vi "Generation Example.vi"() -> ()   [LabVIEW 2025, in "GettingStarted_Gen_148X_Host.lvlib"]
uses:
  GettingStarted_Gen_148X_Host.lvlib
  Common/Types/Serial Channel Configuration.ctl
  <instrlib>/FlexRIO/CSI-2/v2/FPGA/Types/Display Parameters.ctl
  <instrlib>/FlexRIO/CSI-2/v2/Common/Types/LLP Data Type.ctl
  Common/Types/RAW Interpretation for Display.ctl
  <vilib>/userDefined/Silver/nirio_resource_slv.ctl
  <instrlib>/FlexRIO/CSI-2/v2/FPGA/Types/Timestamp ID.ctl
  Common/Types/GPIO Filter.ctl
  Common/Types/Packet Table.ctl
  FPGA/Common/Types/SerDes Identifier.ctl
  <instrlib>/FlexRIO/CSI-2/v2/FPGA/Types/GPIO Bank.ctl
  Common/Types/GPIO Route Configuration.ctl
  Common/Types/GPIO Route Direction.ctl
  Common/Types/GPIO Route Line.ctl
  <vilib>/vision/Image Controls.llb/IMAQ Image.ctl
  <vilib>/Utility/miscctls.llb/LVRowAndColumnUnsignedTypeDef.ctl
  <instrlib>/FlexRIO/API/Host/v1/NI FlexRIO/API/Wait for PoC Safe to Disconnect Channels Array.vi
  <vilib>/FPGAPlugInAG/Dynamic/niLvFpga_Close_Dynamic.vi
  <vilib>/rvi/interface/nirviCloseFPGA/nirviCloseFPGA.xnode
  <instrlib>/FlexRIO/API/Host/v1/NI FlexRIO API v1.lvlib
  Common/GettingStarted_Common_148X_Host.lvlib
  <instrlib>/FlexRIO/CSI-2/v2/FPGA/NI CSI-2 API FPGA v2.lvlib
  FPGA/Common/GettingStarted_Common_148X_FPGA.lvlib
  <instrlib>/FlexRIO/CSI-2/v2/Common/NI CSI-2 API Common v2.lvlib
panel:
  out "Power Over Coax Source In Range":bool[](array[boolean])
  in  "Configuration":T1(tab)
  in  "Display Generated Images":bool=TRUE
  in  "RIO Device":T2="PXI1Slot5"
  in  "Bitfile Path":path=path "C:/dev/hardware-validation/src/labview/auto-vision/Automotive Vision/1487 HIHO GSE/FPGA Bitfiles/PXIe_1487_4_In_4_Out_Gen.lvbitx"
  in  "TDMS File Directory":path=path "C:/dev/hardware-validation/src/labview/auto-vision/Automotive Vision/1487 HIHO GSE/TDMS800x600raw8"
  in  "Log I2C to Disk":bool
  in  "Log GPIO to Disk":bool
  in  "Channel Configurations":T3[](array[typedef])=[{"Serial Channel"="SO1", "FPGA Display Parameters"={"virtual channel"=0.0, "payload data type"=enum."RAW 8", "frame skip count"=0, "line skip count"=0, "pixel skip count"=0.0}, "RAW Display Parameters"={"Interpretation"=enum."Bayer", "Bayer Parameters"={"Pattern"=3, "Algorithm"=0, "Red Gain"=1.0, "Green Gain"=1.0, "Blue Gain"=1.0}}}] {"RAW Display Parameters"."Bayer Parameters"."Blue Gain" min=0.0 max=3.99 step=0.1 format="%_4g"; "RAW Display Parameters"."Bayer Parameters"."Green Gain" min=0.0 max=3.99 step=0.1 format="%_4g"; "RAW Display Parameters"."Bayer Parameters"."Red Gain" min=0.0 max=3.99 step=0.1 format="%_4g"; "RAW Display Parameters"."Bayer Parameters"."Algorithm" items=["Bilinear", "VNG"]; "RAW Display Parameters"."Bayer Parameters"."Pattern" items=["GB", "GR", "BG", "RG"]}
  in  "Serializer (Output) Configuration Script":path=path "C:/dev/hardware-validation/src/labview/auto-vision/Automotive Vision/1487 HIHO GSE/scripts/Image RT Scripts/9295A_RAW8.cpp"
  in  "Packet Timing Error Threshold (s)":dbl=1e-06 format="%#_6p"
  in  "Start Trigger Delay (s)":dbl min=0.0
  out "Actual Serial Output Data Rate (bps)":dbl=-1.0 format="%#_6p"
  in  "Power Over Coax Sink":i32(ring) items=["None"=0, "Auxiliary"=2]
  in  "Reference Clock Frequency (Hz)":dbl=25000000.0 format="%#_6p"
  in  "Requested Serial Ouptut Data Rate (bps)":dbl=-1.0 format="%#_6p"
  in  "Serial Output Active Lane Count":i32(ring)=4 items=["1 Lane"=1, "2 Lanes"=2, "4 Lanes"=4]
  in  "Power Over Coax Source":i32(ring) items=["None", "Internal", "Auxiliary"]
  in  "Timestamp Filter":T7[](array[typedef])
  in  "Enable I2C TAP (All Channels)":bool=TRUE
  in  "GPIO Bank Output Enable":T8
  in  "GPIO Routes":T9[](array[typedef]) {"Serial Channel" max=3 step=1}
  in  "GPIO to Display":T12[](array[typedef])
  in  "GPIO Bank Select":T13
  in  "GPIO Bank Output":T8
  out "GPIO Bank Read":T8
  in  "Update GPIO Output":bool
  in  "Generated Serial Output Channel Data":T14(tab)
  out "Source Rate (fps)(1st Display)":dbl
  out "Update Rate (fps)(1st Display)":dbl
  in  "Serial Channel (1st Display)":fxp<+,3,3>
  out "1st channel display":T15(plugin-control)
  out "Source Rate (fps)(2nd Display)":dbl
  out "Update Rate (fps)(2nd Display)":dbl
  out "2nd channel display":T15(plugin-control)
  in  "Serial Channel (2nd Display)":fxp<+,3,3>
  out "I2C Timestamps":T16
  out "GPIO Timestamps Waveform":digitalwaveform[](graph)
  out "Error Parsing GPIO Timestamps":bool
  out "Generation State":T17(ring)
  out "Number of Generated Packets":u64[](array[numeric])
  out "Packet Timing Errors":bool[](array[boolean])
  out "Waiting for Serializer Setup":bool
  in  "Serializer Setup Complete":bool
  out "Generation Stopped":bool
  out "Power Over Coax Voltage (V)":dbl[](array[numeric]) format="%#.2pV"
  out "Power Over Coax Current (A)":dbl[](array[numeric]) format="%#.2pA"
  out "Power Over Coax Sink In Range":bool[](array[boolean])
  in  "Stop Generation":bool
  out "Error Out":errorcluster
  # "Overview: Configure a generation to replay CSI-2 data and timestamps from disk.\nInstructions: Visit https://ni.com/r/automotive-camera-module-ref for tutorials and reference material on using this example with the PXIe-148X."
  # "Configuration Settings"
  # "Data Output"
  # "Note: Applies to Tap Boards only with\nI2C -> Enable I2C TAP (All Channels) enabled"
  # "Resource Configuration"
  # "Output Configuration"
  # "Channel Configuration"
  # "Power Over Coax Configuration"
  # "Note: Applies to Tap Boards only with\nI2C -> Enable I2C TAP (All Channels) enabled"
  # "Clocking Configuration"
  # "CSI-2 Output Configuration"
  # "Use -1 to request the default data rate"
  # "I2C Timestamp Configuration"
  # "The timestamp filters listed correspond to the I2C traffic for a specific serial channel:\n\nUser24 = SO0\nUser25 = SO1\nUser26 = SO2\nUser27 = SO3\nUser28 = SO4\nUser29 = SO5\nUser30 = SO6\nUser31 = SO7"
  # "I2C TAP Configuration (4 In/4 Out Only)"
  # "GPIO Display Configuration"
  # "GPIO Bank Read / Write Configuration"
  # "GPIO Routing Configuration"
  # "NOTE: Image Display is currently only supported on Windows."
  # "NOTE: Image Display is currently only supported on Windows."
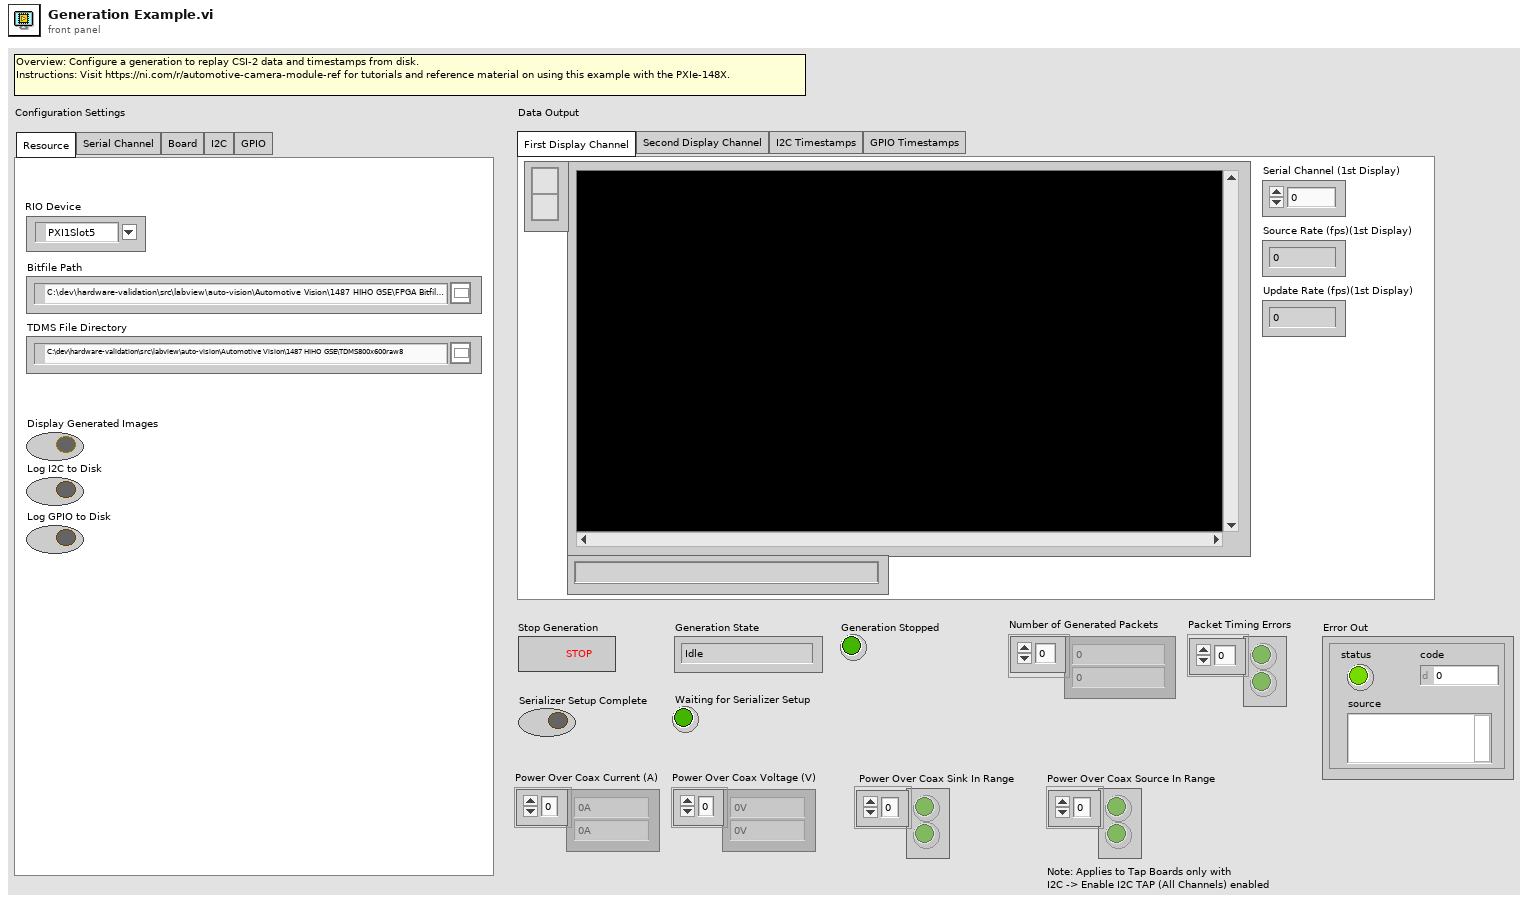
[diagram p1: front panel]
types:
  T1 = enum32{"Resource", "Serial Channel", "Board", "I2C", "GPIO"}
  T2 = typedef "nirio_resource_slv.ctl" = tag
  T3 = typedef "GettingStarted_Common_148X_Host.lvlib/Serial Channel Configuration.ctl" = cluster{"Serial Channel":string, "FPGA Display Parameters":T4, "RAW Display Parameters":cluster{"Interpretation":T6, "Bayer Parameters":cluster{"Pattern":i32, "Algorithm":i32, "Red Gain":dbl, "Green Gain":dbl, "Blue Gain":dbl}}}
  T4 = typedef "NI CSI-2 API FPGA v2.lvlib/Display Parameters.ctl" = cluster{"virtual channel":fxp<+,4,4>, "payload data type":T5, "frame skip count":u16, "line skip count":u8, "pixel skip count":fxp<+,5,5>}
  T5 = typedef "NI CSI-2 API Common v2.lvlib/LLP Data Type.ctl" = enum8{"Frame Start", "Frame End", "Line Start", "Line End", "End of Transmission", "Reserved 0", "Reserved 1", "Reserved 2", "Generic Short Packet 1", "Generic Short Packet 2", "Generic Short Packet 3", "Generic Short Packet 4", "Generic Short Packet 5", "Generic Short Packet 6", "Generic Short Packet 7", "Generic Short Packet 8", "Null", "Blanking Data", "Embedded 8-bit non Image Data", "Generic Long Packet 1", "Generic Long Packet 2", "Generic Long Packet 3", "Generic Long Packet 4", "Reserved 3", "YUV420 8-bit", "YUV420 10-bit", "Legacy YUV420 8-bit", "Reserved 4", "YUV420 8-bit Chroma Shifted", "YUV420 10-bit Chroma Shifted", "YUV422 8-bit", "YUV422 10-bit", "RGB444", "RGB555", "RGB565", "RGB666", "RGB888", "Reserved 5", "Reserved 6", "RAW 24", "RAW 6", "RAW 7", "RAW 8", "RAW 10", "RAW 12", "RAW 14", "RAW 16", "RAW 20", "User Defined 8-bit Data 1", "User Defined 8-bit Data 2", "User Defined 8-bit Data 3", "User Defined 8-bit Data 4", "User Defined 8-bit Data 5", "User Defined 8-bit Data 6", "User Defined 8-bit Data 7", "User Defined 8-bit Data 8", "USL Command", "Reserved 7", "Reserved 8", "Reserved 9", "Reserved 10", "Reserved 11", "Reserved 12", "LRTE EPD Spacer"}
  T6 = typedef "GettingStarted_Common_148X_Host.lvlib/RAW Interpretation for Display.ctl" = enum16{"Grayscale", "Bayer", "RGB", "YUV422", "YUV420", "Legacy YUV420"}
  T7 = typedef "NI CSI-2 API FPGA v2.lvlib/Timestamp ID.ctl" = enum8{"SI0 LLP", "SI1 LLP", "SI2 LLP", "SI3 LLP", "SI4 LLP", "SI5 LLP", "SI6 LLP", "SI7 LLP", "SO0 LLP", "SO1 LLP", "SO2 LLP", "SO3 LLP", "SO4 LLP", "SO5 LLP", "SO6 LLP", "SO7 LLP", "Ser0 GPIO Bank", "Ser1 GPIO Bank", "Ser2 GPIO Bank", "Ser3 GPIO Bank", "Ser4 GPIO Bank", "Ser5 GPIO Bank", "Ser6 GPIO Bank", "Ser7 GPIO Bank", "Des0 GPIO Bank", "Des1 GPIO Bank", "Des2 GPIO Bank", "Des3 GPIO Bank", "Des4 GPIO Bank", "Des5 GPIO Bank", "Des6 GPIO Bank", "Des7 GPIO Bank", "User0", "User1", "User2", "User3", "User4", "User5", "User6", "User7", "User8", "User9", "User10", "User11", "User12", "User13", "User14", "User15", "User16", "User17", "User18", "User19", "User20", "User21", "User22", "User23", "User24", "User25", "User26", "User27", "User28", "User29", "User30", "User31"}
  T8 = typedef "NI CSI-2 API FPGA v2.lvlib/GPIO Bank.ctl" = cluster{"GPIO 0":bool, "GPIO 1":bool, "GPIO 2":bool, "GPIO 3":bool, "GPIO 4":bool, "GPIO 5":bool, "GPIO 6":bool, "GPIO 7":bool, "GPIO 8":bool, "GPIO 9":bool, "GPIO 10":bool}
  T9 = typedef "GettingStarted_Common_148X_Host.lvlib/GPIO Route Configuration.ctl" = cluster{"Direction":T10, "Serial Channel":u8, "Source":T11, "Destination":T11}
  T10 = typedef "GettingStarted_Common_148X_Host.lvlib/GPIO Route Direction.ctl" = enum8{"SO to SI", "SI to SO"}
  T11 = typedef "GettingStarted_Common_148X_Host.lvlib/GPIO Route Line.ctl" = enum16{"GPIO 0", "GPIO 1", "GPIO 2", "GPIO 3", "GPIO 4", "GPIO 5", "GPIO 6", "GPIO 7", "GPIO 8", "GPIO 9", "GPIO 10", "User"}
  T12 = typedef "GettingStarted_Common_148X_Host.lvlib/GPIO Filter.ctl" = cluster{"GPIO Bank":T7, "GPIO Number":i32}
  T13 = typedef "GettingStarted_Common_148X_FPGA.lvlib/SerDes Identifier.ctl" = enum8{"None", "SI 0 Deserializer", "SI 1 Deserializer", "SI 2 Deserializer", "SI 3 Deserializer", "SI 4 Deserializer", "SI 5 Deserializer", "SI 6 Deserializer", "SI 7 Deserializer", "SO 0 Serializer", "SO 1 Serializer", "SO 2 Serializer", "SO 3 Serializer", "SO 4 Serializer", "SO 5 Serializer", "SO 6 Serializer", "SO 7 Serializer", "SI 0 SI 1 Deserializer", "SI 2 SI 3 Deserializer", "SI 4 SI 5 Deserializer", "SI 6 SI 7 Deserializer"}
  T14 = enum32{"First Display Channel", "Second Display Channel", "I2C Timestamps", "GPIO Timestamps"}
  T15 = typedef "IMAQ Image.ctl" = refnum<image>
  T16 = typedef "GettingStarted_Common_148X_Host.lvlib/Packet Table.ctl" = string[][]
  T17 = enum8{"Idle", "Ready For Start Trigger", "Generate Packets", "Done", "Error"}
  T18 = typedef "LVRowAndColumnUnsignedTypeDef.ctl" = cluster{"Row":u32, "Column":u32}
  T19 = typedef "GettingStarted_Common_148X_Host.lvlib/Serial Channel Display Parameters.ctl" = cluster{"images":cluster{"grayscale":T15, "color":T15}, "RAW parameters":cluster{"interpretation":T6, "bayer parameters":cluster{"pattern":i32, "algorithm":i32, "red gain":dbl, "green gain":dbl, "blue gain":dbl}}}
  T20 = typedef "GettingStarted_Gen_148X_Host.lvlib/Channel Source File Paths.ctl" = cluster{"llp packets path":path}
  T21 = cluster{"Source Rate (fps)(1st Display)":refnum<vi>, "Update Rate (fps)(1st Display)":refnum<vi>}
  T22 = cluster{"Source Rate (fps)(2nd Display)":refnum<vi>, "Update Rate (fps)(2nd Display)":refnum<vi>}
  T23 = cluster{"Source Rate (fps)(2nd Display)":refnum<vi>, "Update Rate (fps)(2nd Display)":refnum<vi>}[]
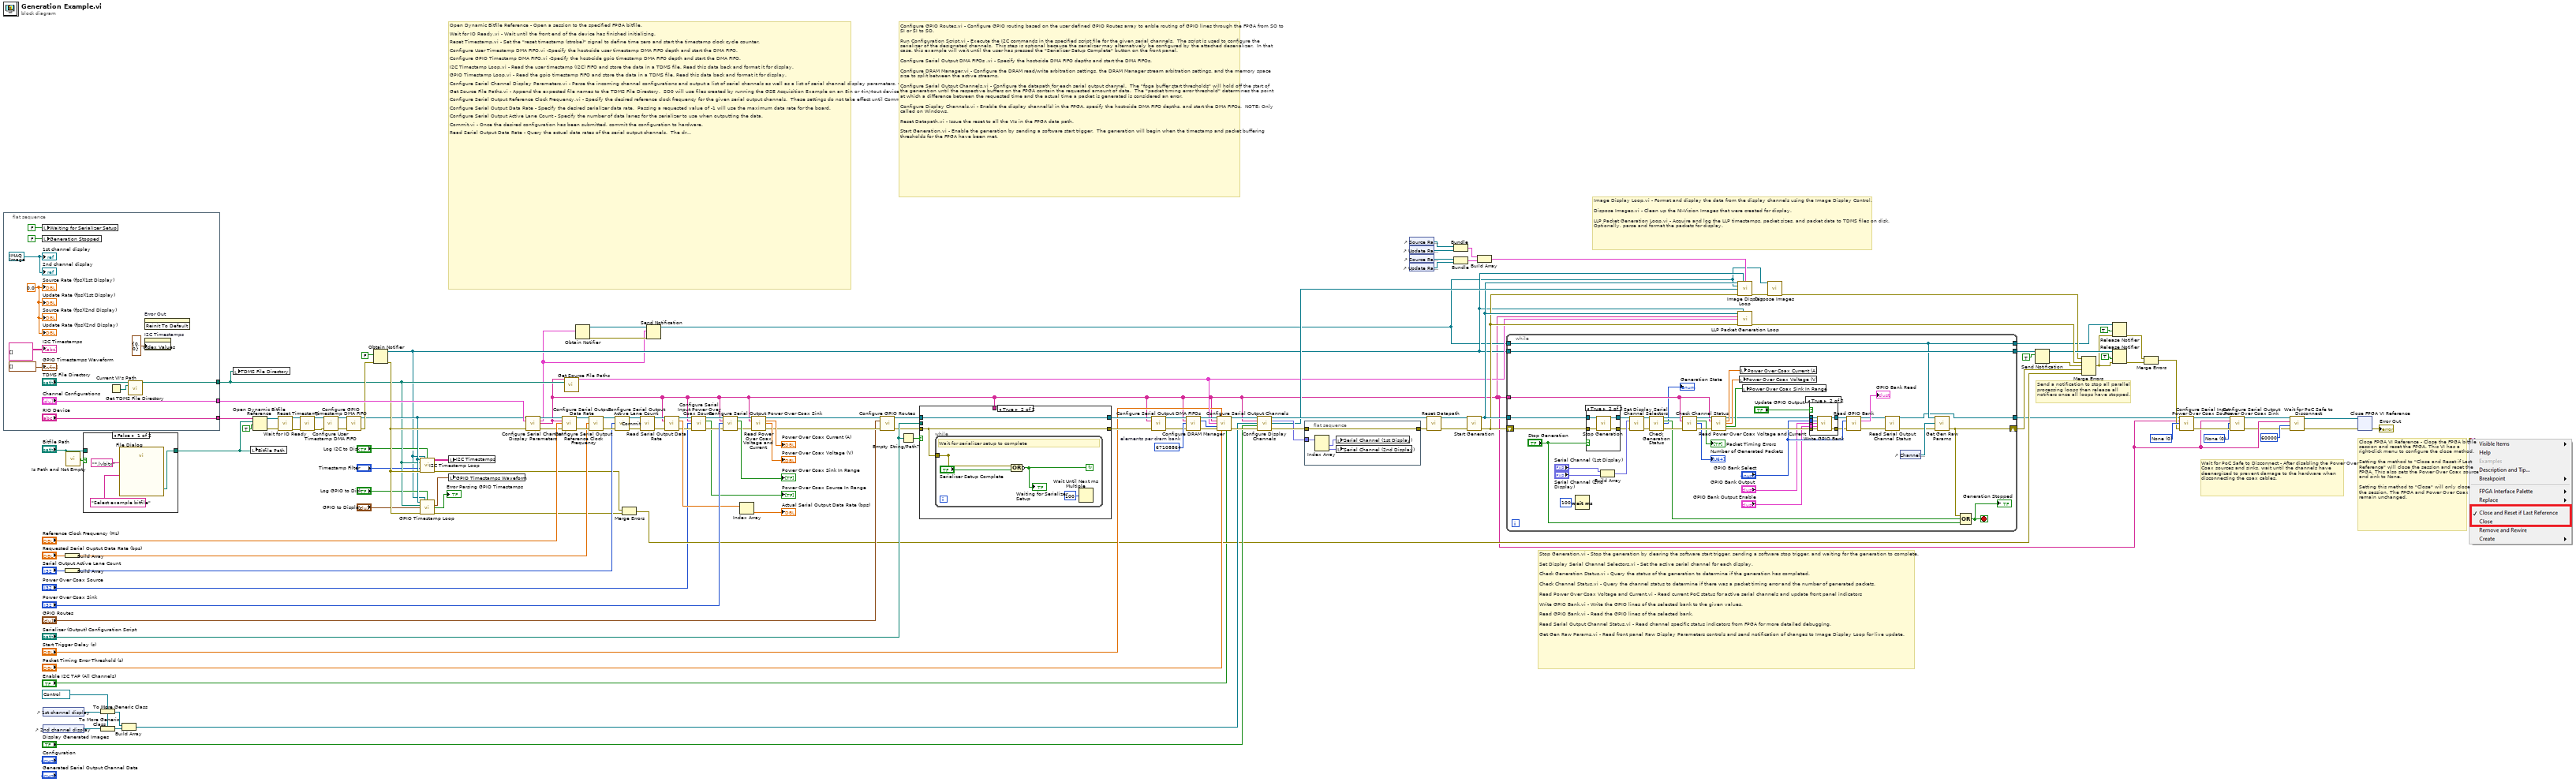
[diagram p0: block diagram]
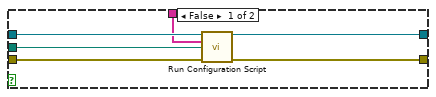
[diagram p2: hidden frame]
diagram:
  w3 = 0 items=["None"=0, "Auxiliary"=2] ("power over coax sink")
  w13 = 0 items=["None", "Internal", "Auxiliary"] ("power over coax source")
  w96 = refnum<vi> refnum ("image display reference")
  w134 = u32 67108864  # elements per dram bank
  # "Wait for PoC Safe to Disconnect - After disabling the Power Over Coax sources and sinks, wait until the channels have deenergized to prevent damage to the hardware when disconnecting the coax cables."
  # "Close FPGA VI Reference - Close the FPGA bitfile session and reset the FPGA. This VI has a right-click menu to configure the close method. \n\nSetting the method to \"Close and Reset if Last Reference\" will close the session and reset the FPGA. This also sets the Power Over Coax source and sink to None.\n\nSetting this method to \"Close\" will only close the session. The FPGA and Power Over Coax remain unchanged."
  # "Send a notification to stop all parallel processing loops then release all notifiers once all loops have stopped."
  # "Image Display Loop.vi - Format and display the data from the display channels using the Image Display Control. \n\nDispose Images.vi - Clean up the NI-Vision Images that were created for display.\n\nLLP Packet Generation Loop.vi - Acquire and log the LLP timestamps, packet sizes, and packet data to TDMS files on disk.  Optionally, parse and format the packets for display."
  # "Stop Generation.vi - Stop the generation by clearing the software start trigger, sending a software stop trigger, and waiting for the generation to complete.\n\nSet Display Serial Channel Selectors.vi - Set the active serial channel for each display.\n\nCheck Generation Status.vi - Query the status of the generation to determine if the generation has completed.\n\nCheck Channel Status.vi - Query the channel status to determine if there was a packet timing error and the number of generated packets.\n\nRead Power Over Coax Voltage and Current.vi - Read current PoC status for active serial channels and update front panel indicators \n\nWrite GPIO Bank.vi - Write the GPIO lines of the selected bank to the given values.\n\nRead GPIO Bank.vi - Read the GPIO lines of the selected bank.\n\nRead Serial Output Channel Status.vi - Read channel specific status indicators from FPGA for more detailed debugging.\n\nGet Gen Raw Params.vi - Read front panel Raw Display Parameters controls and send notification of changes to Image Display Loop for live update."
  # "Configure GPIO Routes.vi - Configure GPIO routing based on the user defined GPIO Routes array to enble routing of GPIO lines through the FPGA from SO to SI or SI to SO. \n\nRun Configuration Script.vi - Execute the I2C commands in the specified script file for the given serial channels.  The script is used to configure the serializer of the designated channels.  This step is optional because the serializer may alternatively be configured by the attached deserializer.  In that case, this example will wait until the user has pressed the \"Serializer Setup Complete\" button on the front panel.\n\nConfigure Serial Output DMA FIFOs .vi - Specify the host-side DMA FIFO depths and start the DMA FIFOs.\n\nConfigure DRAM Manager.vi - Configure the DRAM read/write arbitration settings, the DRAM Manager stream arbitration settings, and the memory space size to split between the active streams.\n\nConfigure Serial Output Channels.vi - Configure the datapath for each serial output channel.  The \"fpga buffer start thresholds\" will hold off the start of the generation until the respective buffers on the FPGA contain the requested amount of data.  The \"packet timing error threshold\" determines the point at which a difference between the requested time and the actual time a packet is generated is considered an error.\n\nConfigure Display Channels.vi - Enable the display channel(s) in the FPGA, specify the host-side DMA FIFO depths, and start the DMA FIFOs.  NOTE: Only called on Windows. \n\nReset Datapath.vi - Issue the reset to all the VIs in the FPGA data path.\n\nStart Generation.vi - Enable the generation by sending a software start trigger.  The generation will begin when the timestamp and packet buffering thresholds for the FPGA have been met."
  # "Open Dynamic Bitfile Reference - Open a session to the specified FPGA bitfile.\n\nWait for IO Ready.vi - Wait until the front end of the device has finished initializing.\n\nReset Timestamp.vi - Set the \"reset timestamp (strobe)\" signal to define time zero and start the timestamp clock cycle counter.\n\nConfigure User Timestamp DMA FIFO.vi -Specify the host-side user timestamp DMA FIFO depth and start the DMA FIFO.\n\nConfigure GPIO Timestamp DMA FIFO.vi -Specify the host-side gpio timestamp DMA FIFO depth and start the DMA FIFO.\n\nI2C Timestamp Loop.vi - Read the user timestamp (I2C) FIFO and store the data in a TDMS file. Read this data back and format it for display.\n\nGPIO Timestamp Loop.vi - Read the gpio timestamp FIFO and store the data in a TDMS file. Read this data back and format it for display.\n\nConfigure Serial Channel Display Parameters.vi - Parse the incoming channel configurations and output a list of serial channels as well as a list of serial channel display parameters, which includes NI-Vision Images and decoding parameters.\n\nGet Source File Paths.vi - Append the expected file names to the TDMS File Directory.  SO0 will use files created by running the GSE Acquisition Example on an 8in or 4in/4out device on channel SI0 (and so on).  Replace this logic if using custom file names.\n\nConfigure Serial Output Reference Clock Frequency.vi - Specify the desired reference clock frequency for the given serial output channels.  These settings do not take effect until Commit.vi is called. \n\nConfigure Serial Output Data Rate - Specify the desired serializer data rate.  Passing a requested value of -1 will use the maximum data rate for the board.\n\nConfigure Serial Output Active Lane Count - Specify the number of data lanes for the serializer to use when outputting the data.\n\nCommit.vi - Once the desired configuration has been submitted, commit the configuration to hardware. \n\nRead Serial Output Data Rate - Query the actual data rates of the serial output channels.  The driver might coerce the data rate to an achievable value\n\nConfigure Serial Input Power Over Coax Source.vi - Specify the source of the power that will be supplied to the devices via the coaxial cables attached to the given serial input channels.  These settings take effect in hardware immediately. Applies to Tap Boards only with I2C -> Enable I2C TAP (All Channels) enabled.\n\nConfigure Serial Output Power Over Coax Sink.vi - Specify whether to sink the power that will be supplied by the devices via the coaxial cables attached to the given serial output channels to the corresponding auxiliary power port.  These settings take effect in hardware immediately.\n\nRead Power Over Coax Voltage and Current.vi - Query the values of the voltage and current detected by the Power over Coax circuitry of the given serial channels."
  n1 = flat-sequence {
    tunnel: ["RIO Device"] -> w118
    tunnel: [w142] -> w41
    tunnel: ["Channel Configurations"] -> w106
    frame #0 {
      w138 = T15 refnum ("1st channel display")
      w139 = 0.0 ("Source Rate (fps)(1st Display)")
      n2 = local write "Waiting for Serializer Setup"(FALSE ("Waiting for Serializer Setup")) -> ()
      n3 = local write "Generation Stopped"(FALSE ("Stopped")) -> ()
      n4 = Current VI's Path() -> (path=w141:path)
      n5 = call "Get TDMS File Directory.vi"("tdms file directory in"="TDMS File Directory", "calling vi path"=w141) -> ("tdms file directory out"=w142:path)  [unwired: 13 in]
      n6 = invoke on="Error Out" class="Clust (strict)" method="Reinit To Default"() -> ()  [unwired: 3 in, 3 out]
      n7 = property on="I2C Timestamps" class="Tbl (strict)"("Index Values"=T18 {"Row"=0, "Column"=0}) -> ()  [unwired: 2 in, 2 out]
      "Update Rate (fps)(1st Display)" <- w139
      "Source Rate (fps)(1st Display)" <- w139
      "Update Rate (fps)(2nd Display)" <- w139
      "Source Rate (fps)(2nd Display)" <- w139
      "1st channel display" <- w138
      "2nd channel display" <- w138
      "I2C Timestamps" <- T16 [] ("I2C Timestamps 2")
      "GPIO Timestamps Waveform" <- digitalwaveform[] [] ("GPIO Timestamps Waveform")
    }
  }
  n8 = control-ref of="1st channel display"() -> (w94:refnum<vi>)
  n9 = control-ref of="2nd channel display"() -> (w95:refnum<vi>)
  n10 = Build Array("Requested Serial Ouptut Data Rate (bps)") -> (w54:dbl[])
  n11 = Build Array("Serial Output Active Lane Count") -> (w52:i32[])
  n12 = call <vilib>:"Is Path and Not Empty.vi"("path"="Bitfile Path") -> ("Is Path and Not Empty?"=w126:bool)  [unwired: 4 in]
  n13 = case shown="False" w126 {
    tunnel: "Bitfile Path" -> [_ w150]
    tunnel: [w148 w150] -> w125
    frame False {
      n14 = call "File Dialog"("prompt"="Select example bitfile", "pattern (all files)"="*.lvbitx") -> ("selected path"=w148:path)  [unwired: 10 in, 3 out]
    }
    frame True {
    }
  }
  n15 = To More Generic Class(target class=w96, reference=w94) -> (generic class reference=w98:refnum<vi>)
  n16 = To More Generic Class(target class=w96, reference=w95) -> (generic class reference=w97:refnum<vi>)
  n17 = Build Array(w98, w97) -> (w85:refnum<vi>[])
  n18 = local write "TDMS File Directory"(w41) -> ()
  n19 = local write "Bitfile Path"(w125) -> ()
  n20 = Open Dynamic Bitfile Reference(0:w118, 1:w125, 2:TRUE ("Run When Loaded")) -> (5:w123:refnum<k20>, 8:w124:errorcluster)  [unwired: 2 in]
  n21 = call <instrlib>:"Wait for IO Ready.vi"("fpga interface in"=w123, "error in"=w124) -> ("fpga interface out"=w78:refnum<k20>, "error out"=w77:errorcluster)  [unwired: 10 in, 2 out]
  n22 = call "Reset Timestamp.vi"("fpga interface in"=w78, "error in (no error)"=w77) -> ("fpga interface out"=w50:refnum<k20>, "error out"=w48:errorcluster)  [unwired: 16 in]
  n23 = call "Configure User Timestamp DMA FIFO.vi"("fpga interface in"=w50, "error in (no error)"=w48) -> ("fpga interface out"=w49:refnum<k20>, "error out"=w47:errorcluster)  [unwired: 12 in]
  n24 = call "Configure GPIO Timestamp DMA FIFO.vi"("fpga interface in"=w49, "error in (no error)"=w47) -> ("fpga interface out"=w44:refnum<k20>, "error out"=w46:errorcluster)  [unwired: 12 in]
  n25 = Obtain Notifier(notification data type=FALSE ("result"), error in (no error)=w46) -> (notifier out=w30:refnum<notifier>, error out=w45:errorcluster)  [unwired: 2 in, 1 out]
  n26 = call "I2C Timestamp Loop.vi"("fpga interface in"=w44, "'stop' notifier"=w30, "log i2c to disk"="Log I2C to Disk", "tdms file directory"=w41, "timestamp filter"="Timestamp Filter", "error in (no error)"=w45) -> ("i2c data"=w39:string[][], "error out"=w43:errorcluster)  [unwired: 8 in]
  n27 = call "GPIO Timestamp Loop.vi"("fpga interface in"=w44, "'stop' notifier"=w30, "log gpio to disk"="Log GPIO to Disk", "tdms file directory"=w41, "gpio to display"="GPIO to Display", "error in (no error)"=w45) -> ("gpio timestamps waveform"=w38:digitalwaveform[], "error parsing gpio timestamps"=→"Error Parsing GPIO Timestamps":bool, "error out"=w42:errorcluster)  [unwired: 7 in]
  n28 = local write "I2C Timestamps"(w39) -> ()
  n29 = local write "GPIO Timestamps Waveform"(w38) -> ()
  n30 = call "Configure Serial Channel Display Parameters.vi"("fpga interface in"=w44, "serial channel configurations"=w106, "error in (no error)"=w45) -> ("fpga interface out"=w107:refnum<k20>, "serial channel display parameters"=w27:T19[], "serial channels"=w4:string[], "error out"=w108:errorcluster)  [unwired: 9 in]
  n31 = call "Configure Serial Output Reference Clock Frequency.vi"("fpga interface in"=w107, "serial output channels"=w4, "serial output reference clock frequency (Hz)"="Reference Clock Frequency (Hz)", "error in (no error)"=w108) -> ("fpga interface out"=w65:refnum<k20>, "error out"=w64:errorcluster)  [unwired: 10 in]
  n32 = call "Get Source File Paths.vi"("serial output channels"=w4, "base tdms file path"=w41) -> ("source file paths"=w76:T20[])  [unwired: 13 in]
  n33 = Obtain Notifier(notification data type=w27) -> (notifier out=w29:refnum<notifier>, error out=w28:errorcluster)  [unwired: 3 in, 1 out]
  n34 = call "Configure Serial Output Data Rate.vi"("fpga interface in"=w65, "serial output data rates"=w54, "error in (no error)"=w64) -> ("fpga interface out"=w62:refnum<k20>, "error out"=w63:errorcluster)  [unwired: 11 in]
  n35 = call "Configure Serial Output Active Lane Count.vi"("fpga interface in"=w62, "serial output active lane counts"=w52, "error in (no error)"=w63) -> ("fpga interface out"=w61:refnum<k20>, "error out"=w60:errorcluster)  [unwired: 11 in]
  n36 = Merge Errors(w43, w42) -> (w31:errorcluster)
  n37 = call <instrlib>:"Commit.vi"("fpga interface in"=w61, "error in"=w60) -> ("fpga interface out"=w58:refnum<k20>, "error out"=w59:errorcluster)  [unwired: 12 in]
  n38 = Send Notification(notification=w27, notifier=w29, error in (no error)=w28) -> (notifier out=w26:refnum<notifier>)  [unwired: 1 out]
  n39 = call "Read Serial Output Data Rate.vi"("fpga interface in"=w58, "serial output channels"=w4, "error in (no error)"=w59) -> ("fpga interface out"=w19:refnum<k20>, "serial output data rates (bps)"=w57:dbl[], "error out"=w20:errorcluster)  [unwired: 10 in]
  n40 = call "Configure Serial Input Power Over Coax Source.vi"("fpga interface in"=w19, "serial input channels"=w4, "power over coax source"="Power Over Coax Source", "error in (no error)"=w20) -> ("fpga interface out"=w18:refnum<k20>, "power over coax source in range"=→"Power Over Coax Source In Range":bool[], "error out"=w17:errorcluster)  [unwired: 9 in]
  n41 = call "Configure Serial Output Power Over Coax Sink.vi"("fpga interface in"=w18, "serial output channels"=w4, "power over coax sink"="Power Over Coax Sink", "error in (no error)"=w17) -> ("fpga interface out"=w121:refnum<k20>, "power over coax sink in range"=→"Power Over Coax Sink In Range":bool[], "error out"=w122:errorcluster)  [unwired: 9 in]
  n42 = Index Array(array=w57) -> (element=→"Actual Serial Output Data Rate (bps)":dbl)  [unwired: 1 in]
  n43 = call "Read Power Over Coax Voltage and Current.vi"("fpga interface in"=w121, "serial channels"=w4, "error in (no error)"=w122) -> ("fpga interface out"=w81:refnum<k20>, "current (A)"=→"Power Over Coax Current (A)":dbl[], "voltage (V)"=→"Power Over Coax Voltage (V)":dbl[], "error out"=w80:errorcluster)  [unwired: 8 in, 1 out]
  n44 = call "Configure GPIO Routes.vi"("fpga interface in"=w81, "gpio routes"="GPIO Routes", "error in (no error)"=w80) -> ("fpga interface out"=w75:refnum<k20>, "error out"=w74:errorcluster)  [unwired: 11 in]
  n45 = Empty String/Path?(string/path="Serializer (Output) Configuration Script") -> (empty?=w112:bool)
  n46 = case shown="True" w112 {
    tunnel: [w156 w157] -> w133
    tunnel: "Serializer (Output) Configuration Script" -> [w155 _]
    tunnel: [w154 w158] -> w129
    tunnel: w74 -> [w153 w157]
    tunnel: w75 -> [w152 w158]
    tunnel: w4 -> [w151 _]
    frame False {
      n47 = call "Run Configuration Script.vi"("fpga interface in"=w152, "serial channels"=w151, "configuration script"=w155, "error in (no error)"=w153) -> ("fpga interface out"=w154:refnum<k20>, "error out"=w156:errorcluster)  [unwired: 10 in]
    }
    frame True {
      n48 = while {
        tunnel: w157 -> [w159]
        tunnel: [w159] -> _
        stop <- w160 continue-if-true
        # "Wait for serializer setup to complete"
        n49 = Compound Arithmetic op=OR(w159, "Serializer Setup Complete") -> (invert w160:bool)
        "Waiting for Serializer Setup" <- w160
        n50 = Wait Until Next ms Multiple(millisecond multiple=u32 100) -> ()  [unwired: 1 out]
      }
    }
  }
  n51 = call "Configure Serial Output DMA FIFOs.vi"("fpga interface in"=w129, "serial output channels"=w4, "error in (no error)"=w133) -> ("fpga interface out"=w114:refnum<k20>, "error out"=w113:errorcluster)  [unwired: 11 in]
  n52 = call "Configure DRAM Manager.vi"("fpga interface in"=w114, "serial output channels"=w4, "elements per dram bank"=w134, "error in (no error)"=w113) -> ("fpga interface out"=w115:refnum<k20>, "dram partition sizes (bytes)"=w109:u64[], "error out"=w116:errorcluster)  [unwired: 9 in]
  n53 = call "Configure Serial Output Channels.vi"("fpga interface in"=w115, "start trigger delay (s)"="Start Trigger Delay (s)", "serial output channels"=w4, "source file paths"=w76, "dram partition sizes (bytes)"=w109, "error in (no error)"=w116, "packet timing error threshold (s)"="Packet Timing Error Threshold (s)", "enable i2c tap (all channels)"="Enable I2C TAP (All Channels)") -> ("fpga interface out"=w90:refnum<k20>, "error out"=w89:errorcluster)  [unwired: 6 in]
  n54 = call "Configure Display Channels.vi"("fpga interface in"=w90, "serial channels"=w4, "display references in"=w85, "enable image display"="Display Generated Images", "error in (no error)"=w89) -> ("fpga interface out"=w91:refnum<k20>, "display serial channels"=w87:fxp<+,3,3>[], "display references out"=w86:refnum<vi>[], "error out"=w88:errorcluster)  [unwired: 7 in]
  n55 = flat-sequence {
    tunnel: w87 -> [w164]
    tunnel: w88 -> [w163]
    tunnel: [w163] -> w99
    frame #0 {
      n56 = Index Array(array=w164) -> (element #1=w166:fxp<+,3,3>, element #2=w165:fxp<+,3,3>)  [unwired: 2 in]
      n57 = local write "Serial Channel (1st Display)"(w166) -> ()
      n58 = local write "Serial Channel (2nd Display)"(w165) -> ()
    }
  }
  n59 = control-ref of="Source Rate (fps)(1st Display)"() -> (w100:refnum<vi>)
  n60 = control-ref of="Update Rate (fps)(1st Display)"() -> (w101:refnum<vi>)
  n61 = control-ref of="Source Rate (fps)(2nd Display)"() -> (w102:refnum<vi>)
  n62 = control-ref of="Update Rate (fps)(2nd Display)"() -> (w103:refnum<vi>)
  n63 = call "Reset Datapath.vi"("fpga interface in"=w91, "error in (no error)"=w99) -> ("fpga interface out"=w132:refnum<k20>, "error out"=w51:errorcluster)  [unwired: 12 in]
  n64 = Bundle("Source Rate (fps)(1st Display)"=w100, "Update Rate (fps)(1st Display)"=w101) -> (w105:T21)  [unwired: 1 in]
  n65 = Bundle("Source Rate (fps)(2nd Display)"=w102, "Update Rate (fps)(2nd Display)"=w103) -> (w104:T22)  [unwired: 1 in]
  n66 = call "Start Generation.vi"("fpga interface in"=w132, "error in (no error)"=w51) -> ("fpga interface out"=w84:refnum<k20>, "error out"=w83:errorcluster)  [unwired: 12 in]
  n67 = Build Array(w105, w104) -> (w92:T23)
  n68 = while {
    shift-right: [w172] -> w32
    shift-left: w83 -> [w175]
    tunnel: w84 -> [w193]
    tunnel: [w168] -> w7
    tunnel: w4 -> [w200]
    tunnel: [w174] -> w70
    tunnel: w30 -> [w174]
    tunnel: w26 -> [w171]
    tunnel: [w171] -> w25
    stop <- w176 stop-if-true
    n69 = Wait (ms)(milliseconds to wait=u32 100) -> ()  [unwired: 1 out]
    n70 = case shown="True" "Stop Generation" {
      tunnel: [w218 w222] -> w186
      tunnel: w175 -> [w218 w221]
      tunnel: [w217 w220] -> w189
      tunnel: w193 -> [w217 w219]
      frame False {
      }
      frame True {
        n71 = call "Stop Generation.vi"("fpga interface in"=w219, "error in (no error)"=w221) -> ("fpga interface out"=w220:refnum<k20>, "error out"=w222:errorcluster)  [unwired: 12 in]
      }
    }
    n72 = Build Array("Serial Channel (1st Display)", "Serial Channel (2nd Display)") -> (w190:fxp<+,3,3>[])
    n73 = call "Set Display Serial Channel Selectors.vi"("fpga interface in"=w189, "display serial channel selectors"=w190, "error in (no error)"=w186) -> ("fpga interface out"=w188:refnum<k20>, "error out"=w187:errorcluster)  [unwired: 11 in]
    n74 = call "Check Generation Status.vi"("fpga interface in"=w188, "error in (no error)"=w187) -> ("fpga interface out"=w196:refnum<k20>, "generation done"=w195:bool, "generation state"=→"Generation State":T17, "error out"=w197:errorcluster)  [unwired: 10 in]
    n75 = call "Check Channel Status.vi"("fpga interface in"=w196, "serial output channels"=w200, "error in (no error)"=w197) -> ("fpga interface out"=w202:refnum<k20>, "packet timing errors"=→"Packet Timing Errors":bool[], "number of generated packets"=→"Number of Generated Packets":u64[], "error out"=w201:errorcluster)  [unwired: 9 in]
    n76 = call "Read Power Over Coax Voltage and Current.vi"("fpga interface in"=w202, "serial channels"=w200, "error in (no error)"=w201) -> ("fpga interface out"=w179:refnum<k20>, "current (A)"=w205:dbl[], "voltage (V)"=w203:dbl[], "in range"=w204:bool[], "error out"=w207:errorcluster)  [unwired: 8 in]
    n77 = local write "Power Over Coax Voltage (V)"(w203) -> ()
    n78 = local write "Power Over Coax Current (A)"(w205) -> ()
    n79 = local write "Power Over Coax Sink In Range"(w204) -> ()
    n80 = case shown="True" "Update GPIO Output" {
      tunnel: w179 -> [w209 w216]
      tunnel: w207 -> [w208 w215]
      tunnel: "GPIO Bank Output" -> [_ w214]
      tunnel: [w209 w213] -> w181
      tunnel: [w208 w212] -> w182
      tunnel: "GPIO Bank Select" -> [_ w211]
      tunnel: "GPIO Bank Output Enable" -> [_ w210]
      frame False {
      }
      frame True {
        n81 = call "Write GPIO Bank.vi"("fpga interface in"=w216, "gpio bank select"=w211, "gpio bank output"=w214, "gpio bank output enable"=w210, "error in (no error)"=w215) -> ("fpga interface out"=w213:refnum<k20>, "error out"=w212:errorcluster)  [unwired: 9 in]
      }
    }
    n82 = call "Read GPIO Bank.vi"("fpga interface in"=w181, "gpio bank select"="GPIO Bank Select", "error in (no error)"=w182) -> ("fpga interface out"=w170:refnum<k20>, "gpio bank output"=→"GPIO Bank Read":T8, "error out"=w169:errorcluster)  [unwired: 10 in]
    n83 = call "Read Serial Output Channel Status.vi"("fpga interface in"=w170, "error in (no error)"=w169) -> ("fpga interface out"=w168:refnum<k20>, "error out"=w167:errorcluster)  [unwired: 11 in, 1 out]
    n84 = control-ref of="Channel Configurations"() -> (w173:refnum<vi>)
    n85 = call "Get Gen Raw Params.vi"("raw display notifier"=w171, "Channel Configurations"=w173, "error in (no error)"=w167) -> ("error out"=w172:errorcluster)  [unwired: 12 in]
    n86 = Compound Arithmetic op=OR(w172, w195, "Stop Generation") -> (w176:bool)
    "Generation Stopped" <- w176
  }
  n87 = call "Image Display Loop.vi"("fpga interface in"=w84, "'stop' notifier"=w30, "rate references"=w92, "raw display notifier"=w26, "display references"=w86, "error in (no error)"=w83) -> ("error out"=w93:errorcluster)  [unwired: 9 in]
  n88 = call "LLP Packet Generation Loop.vi"("fpga interface in"=w84, "'stop' notifier"=w30, "serial channels"=w4, "source file paths"=w76, "error in"=w83) -> ("error out"=w71:errorcluster)  [unwired: 10 in]
  n89 = call "Dispose Images.vi"("raw display notifier"=w26, "error in (no error)"=w93) -> ("error out"=w40:errorcluster)  [unwired: 13 in]
  n90 = Send Notification(notification=TRUE, notifier=w70) -> (notifier out=w68:refnum<notifier>, error out=w66:errorcluster)  [unwired: 1 in]
  n91 = Merge Errors(w40, w71, w66, w32, w31) -> (w23:errorcluster)
  n92 = Release Notifier(notifier=w25, force destroy? (F)=TRUE, error in (no error)=w23) -> (error out=w22:errorcluster)  [unwired: 2 out]
  n93 = Release Notifier(notifier=w68, force destroy? (F)=TRUE, error in (no error)=w23) -> (error out=w21:errorcluster)  [unwired: 2 out]
  n94 = Merge Errors(w22, w21) -> (w8:errorcluster)
  n95 = call "Configure Serial Input Power Over Coax Source.vi"("fpga interface in"=w7, "serial input channels"=w4, "power over coax source"=w13, "error in (no error)"=w8) -> ("fpga interface out"=w5:refnum<k20>, "error out"=w6:errorcluster)  [unwired: 9 in, 1 out]
  n96 = call "Configure Serial Output Power Over Coax Sink.vi"("fpga interface in"=w5, "serial output channels"=w4, "power over coax sink"=w3, "error in (no error)"=w6) -> ("fpga interface out"=w1:refnum<k20>, "error out"=w2:errorcluster)  [unwired: 9 in, 1 out]
  n97 = call-poly <instrlib>:"Wait for PoC Safe to Disconnect.vi"("error in"=w2, "Timeout (ms)"=60000 ("Wait for Safe to Disconnect Timeout (ms)"), "Channels"=w4, "fpga interface in"=w1) -> ("error out"=w11:errorcluster, "fpga interface out"=w10:refnum<k20>)  [unwired: 6 in]
  n98 = xnode ("Close FPGA VI Reference")("FPGA VI Reference In"=w10, "error in"=w11) -> ("error out"=→"Error Out":errorcluster)
